vi "Check Status of Home Routine.vi"(8 "error in (no error)":errorcluster, 11 "FINE SIM Motion Axis":refnum<class "FINE SIM Motion Axis.lvclass">) -> (0 "error out":errorcluster, 3 "FINE SIM Motion Axis":refnum<class "FINE SIM Motion Axis.lvclass">)   [LabVIEW 2022 SP3, in "FINE SIM Motion Axis.lvclass"]
uses:
  FINE SIM Motion Axis.lvclass
  FINE SIM Motion Axis.lvclass/FINE SIM Motion Axis.ctl
  TypeDefs/Homing Status.ctl
  Accessors/Read Sim Axis Data.vi
  Accessors/Write Sim Axis Data.vi
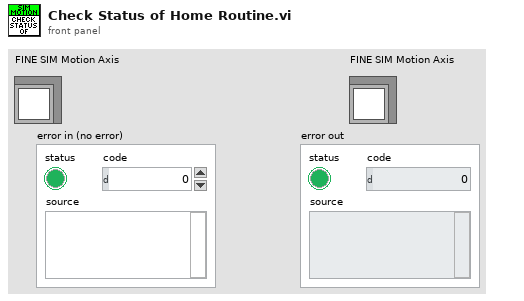
[diagram p1: front panel]
types:
  T1 = typedef "FINE SIM Motion Axis.lvclass/Axis Data.ctl" = cluster{"Axis Parameters":T2, "Time Stamp":timestamp, "Settings":T4}
  T2 = typedef "FINE SIM Motion Axis.lvclass/Axis Parameters.ctl" = cluster{"Moving":bool, "Homed":bool, "Desired Position":dbl, "Current Positon":dbl, "Current Speed":dbl, "Home Status":T3}
  T3 = typedef "FINE SIM Motion Axis.lvclass/Homing Status.ctl" = enum16{"Idle", "Inital Home Motion", "Final Home Motion", "Done Homing"}
  T4 = typedef "FINE SIM Motion Axis.lvclass/Settings.ctl" = cluster{"Axis Name":string, "Axis Settings":T5}
  T5 = typedef "FINE SIM Motion Axis.lvclass/Axis Settings.ctl" = cluster{"Speed":dbl, "Acceleration":dbl}
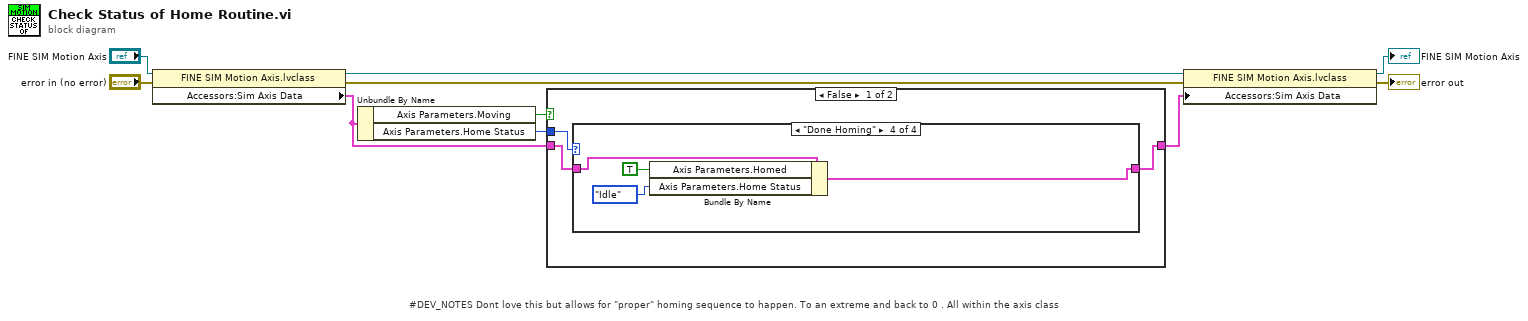
[diagram p0: block diagram]
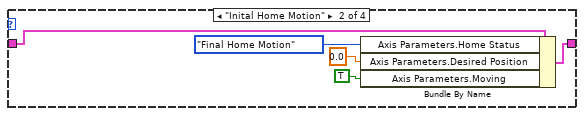
[diagram p3: hidden frame]
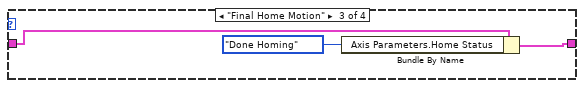
[diagram p4: hidden frame]
diagram:
  # "#DEV_NOTES Dont love this but allows for \"proper\" homing sequence to happen. To an extreme and back to 0 . All within the axis class"
  n1 = property class="FINE SIM Motion Axis.lvclass"(reference="FINE SIM Motion Axis", error in="error in (no error)") -> (reference out=w5:refnum<class "FINE SIM Motion Axis.lvclass">, error out=w8:errorcluster, "Accessors:Sim Axis Data"=w3:T1)
  n2 = Unbundle By Name(w3) -> ("Axis Parameters.Moving"=w7:bool, "Axis Parameters.Home Status"=w9:T3)
  n3 = case shown="False" w7 {
    tunnel: w9 -> [w11 _]
    tunnel: [w13 w27] -> w4
    tunnel: w3 -> [w12 w27]
    frame False {
      n4 = case shown="\"Done Homing\"" w11 {
        tunnel: [w14 w18 w22 w26] -> w13
        tunnel: w12 -> [w14 w15 w21 w25]
        frame "Idle" {
        }
        frame "Inital Home Motion" {
          n5 = Bundle By Name(cluster=w15, "Axis Parameters.Home Status"=Homing_Status."Final Home Motion", "Axis Parameters.Desired Position"=0.0, "Axis Parameters.Moving"=TRUE) -> (w18:T1)
        }
        frame "Final Home Motion" {
          n6 = Bundle By Name(cluster=w21, "Axis Parameters.Home Status"=Homing_Status."Done Homing") -> (w22:T1)
        }
        frame "Done Homing" {
          n7 = Bundle By Name(cluster=w25, "Axis Parameters.Homed"=TRUE, "Axis Parameters.Home Status"=Homing_Status."Idle") -> (w26:T1)
        }
      }
    }
    frame True {
    }
  }
  n8 = property class="FINE SIM Motion Axis.lvclass"(reference=w5, error in=w8, "Accessors:Sim Axis Data"=w4) -> (reference out=→"FINE SIM Motion Axis":refnum<class "FINE SIM Motion Axis.lvclass">, error out=→"error out":errorcluster)
